vi "myRIO_BRig_RT__Case_Exp_State_Timeout.vi"(4 "input_dataLC":u16[](array[numeric]), 6 "input_LC":bool, 10 "input_state":T1, 11 "input_dataCurrent":u16[](array[numeric])) -> (0 "output_LC":bool, 2 "output_state":T1, 3 "output_dataCurrent":u16[](array[numeric]))   [LabVIEW 2014]
uses:
  myRIO_BRig_RT__Case_Exp_stateList.ctl
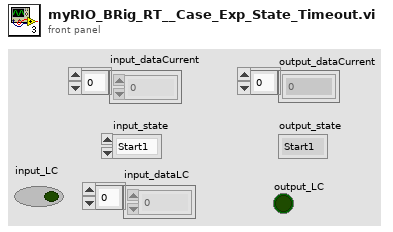
[diagram p1: front panel]
types:
  T1 = typedef "myRIO_BRig_RT__Case_Exp_stateList.ctl" = enum16{"Start1", "Start2", "Start3", "saveSettings1", "saveSettings2", "saveSettings3", "saveSettings4", "saveSettings_LC_ENL_l1", "saveSettings_LC_ENL_l2", "saveSettings_LC_Cue_l1", "saveSettings_LC_Cue_l2", "saveSettings6_LC_l1_Other", "SaveSettings6_LC_l2_Other", "setSettings_Audio", "setSettings_Laser", "initBlock_pre", "initBlock", "initBlock2", "initBlock_post", "initTrial_pre", "initTrial", "initTrial2", "initTrial3", "initTrial4", "initTrial_LC_ENL1", "initTrial_LC_Cue1", "initTrial_LC_Cue1_2", "initTrial_LC_Sel", "initTrial_post", "ENL1_pre", "ENL1", "ENL1_post", "ENL1Penalty_pre", "ENL1Penalty", "ENL2_pre", "ENL2", "ENL2Penalty_pre", "ENL2Penalty", "Cue1_pre", "Cue1", "Cue1_post", "Cue1Penalty_pre", "Cue1Penalty", "Cue2_pre", "Cue2", "Cue2Penalty_pre", "Cue2Penalty", "Selection_pre", "Selection", "Select_post", "SelectReward_pre", "SelectReward", "SelectRewardPost_pre", "SelectRewardPost", "SelectWrong_pre", "SelectWrong", "SelectWrong_post", "SelectTimeout_pre", "SelectTimeout", "SelectTimeout_post", "endTrial_pre", "endTrial1", "endTrial2", "endTrial3", "endTrial_post", "endBlock_pre", "endBlock", "endBlock_post", "endExp", "commConnect", "commUpload_pre", "commUpload_dataBlock", "commUpload_dataCurrent", "commUpload_dataExp", "commUpload_dataLC", "commUpload_dataTrial", "commUpload_post", "saveData_pre", "saveData_dataBlock", "saveData_dataCurrent", "saveData_dataExp", "saveData_dataLC", "saveData_dataTrial", "saveData_post", "empty_endBlock1", "empty_endBlock2", "empty_endTrial1", "empty_endTrial2", "empty_endTrial3", "empty_endTrial4", "empty_endTrial5", "dummyState", "dummyState_endBlock"}
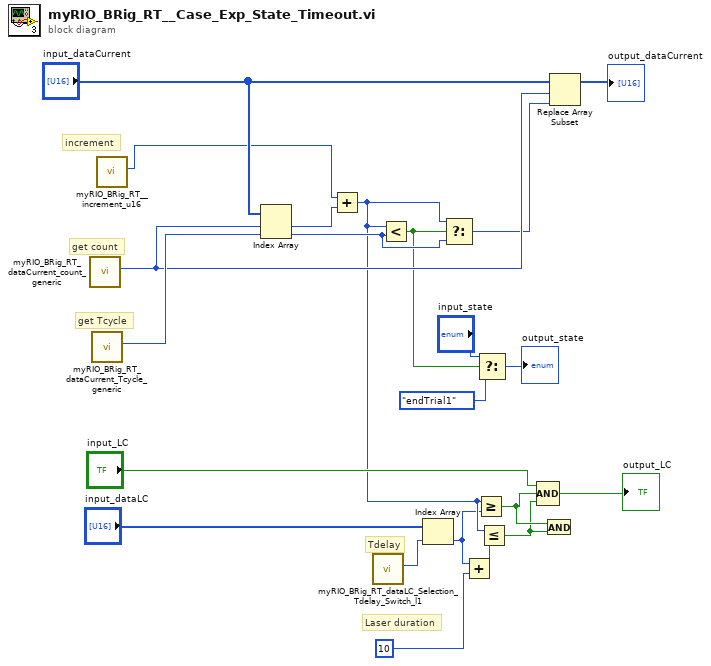
[diagram p0: block diagram]
diagram:
  # "Laser duration"
  # "Tdelay"
  # "increment"
  # "get Tcycle"
  # "get count"
  n1 = call "myRIO_BRig_RT_dataCurrent_count_generic.vi"() -> ("output_count_generic"=w18:i32)  [unwired: 11 in]
  n2 = call "myRIO_BRig_RT_dataCurrent_Tcycle_generic.vi"() -> ("output_Tcycle_generic"=w20:i32)  [unwired: 11 in]
  n3 = call "myRIO_BRig_RT__increment_u16.vi"() -> ("output_increment__u16"=w14:u16)  [unwired: 11 in]
  n4 = Index Array(array="input_dataCurrent", index #1=w18, index #2=w20) -> (element #1=w19:u16, element #2=w17:u16)
  n5 = Add(x=w14, y=w19) -> (x+y=w6:u16)
  n6 = call "myRIO_BRig_RT_dataLC_Selection_Tdelay_Switch_l1.vi"() -> ("output_Selection_Tdelay_Switch_l1"=w13:i32)  [unwired: 11 in]
  n7 = Less?(x=w6, y=w17) -> (x < y?=w15:bool)
  n8 = Index Array(array="input_dataLC", index=w13) -> (element=w5:u16)
  n9 = Select(t=w6, s=w15, f=w17) -> (s? t:f=w16:u16)
  n10 = Add(x=w5, y=u16 10) -> (x+y=w4:u16)
  n11 = Greater Or Equal?(x=w6, y=w5) -> (x >= y?=w2:bool)
  n12 = Select(t="input_state", s=w15, f=myRIO_BRig_RT__Case_Exp_stateList."endTrial1" ("Enum")) -> (s? t:f=→"output_state":T1)
  n13 = Less Or Equal?(x=w6, y=w4) -> (x <= y?=w1:bool)
  n14 = Compound Arithmetic op=AND("input_LC", w2, w1) -> (→"output_LC":bool)
  n15 = And(x=w2, y=w1) -> ()  [unwired: 1 out]
  n16 = Replace Array Subset(array="input_dataCurrent", new element=w16, index=w18) -> (→"output_dataCurrent":u16[])
